vi "Motor_log_filename.vi"(11 "File Path Control":path) -> (2 "Motor log file name (full path)":path, 3 "Motor log filename":string)   [LabVIEW 2012]
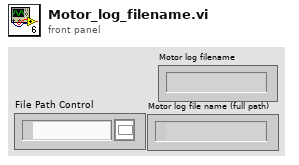
[diagram p1: front panel]
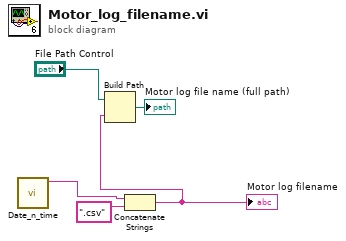
[diagram p0: block diagram]
diagram:
  n1 = call "Date_n_time.vi"() -> ("date string"=w5:string)  [unwired: 9 in, 2 out]
  n2 = Concatenate Strings(w5, ".csv" ("name or relative path")) -> (w2:string)
  "Motor log filename" <- w2
  n3 = Build Path(base path="File Path Control", name or relative path=w2) -> (appended path=→"Motor log file name (full path)":path)
